vi "VisionTotal.vi"   [LabVIEW 2016]
uses:
  Robot Global Data.vi
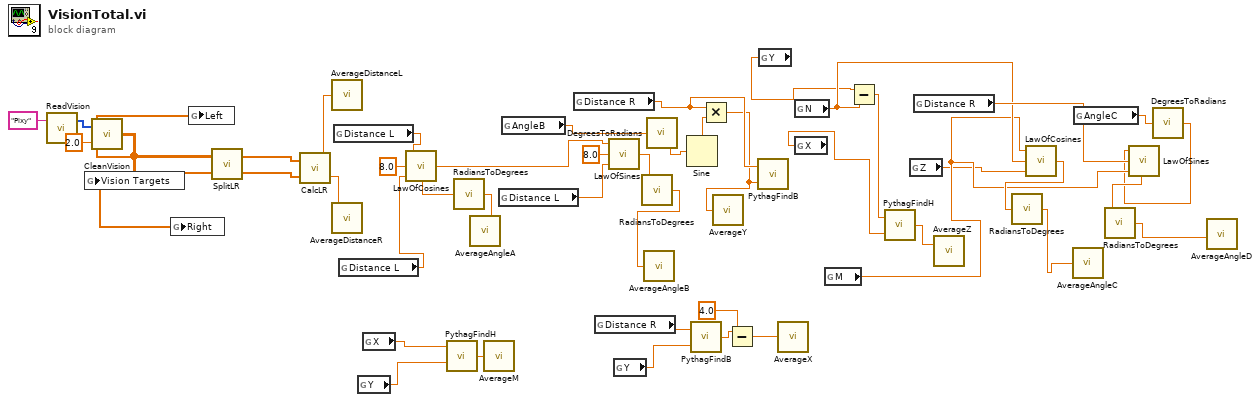
[diagram p0: block diagram]
diagram:
  n1 = call "ReadVision.vi"("Name"="Pixy") -> ("Target Data"=w42:u16[])  [unwired: 2 in]
  n2 = call "CleanVision.vi"("Targets"=2.0, "Input"=w42) -> ("Output"=w41:dbl[][])
  n3 = global write "Robot Global Data.vi" "Vision Targets"(w41) -> ()
  n4 = call "SplitLR.vi"("Vision Targets"=w41) -> ("Right"=w39:dbl[], "Left"=w40:dbl[])  [unwired: 1 in]
  n5 = global write "Robot Global Data.vi" "Right"(w39) -> ()
  n6 = global write "Robot Global Data.vi" "Left"(w40) -> ()
  n7 = call "CalcLR.vi"("Right"=w39, "Left"=w40) -> ("Right"=w25:dbl, "Left"=w24:dbl)
  n8 = call "AverageDistanceL.vi"("Input"=w24) -> ()  [unwired: 1 in]
  n9 = call "AverageDistanceR.vi"("Input"=w25) -> ()  [unwired: 1 in]
  n10 = global read "Robot Global Data.vi" "Distance L"() -> (w12:dbl)
  n11 = global read "Robot Global Data.vi" "Distance L"() -> (w11:dbl)
  n12 = global read "Robot Global Data.vi" "Y"() -> (w1:dbl)
  n13 = global read "Robot Global Data.vi" "X"() -> (w2:dbl)
  n14 = call "LawOfCosines.vi"("Right"=w11, "Opposite"=8.0, "Left"=w12) -> ("Angle"=w35:dbl)
  n15 = call "PythagFindH.vi"("Side B"=w1, "Side A"=w2) -> ("Side H"=w3:dbl)
  n16 = call "RadiansToDegrees.vi"("Radians"=w35) -> ("Degrees"=w23:dbl)
  n17 = call "AverageAngleA.vi"("Input"=w23) -> ()  [unwired: 1 in]
  n18 = call "AverageM.vi"("Input"=w3) -> ()  [unwired: 1 in]
  n19 = global read "Robot Global Data.vi" "Distance L"() -> (w37:dbl)
  n20 = global read "Robot Global Data.vi" "AngleB"() -> (w22:dbl)
  n21 = global read "Robot Global Data.vi" "Distance R"() -> (w34:dbl)
  n22 = global read "Robot Global Data.vi" "Distance R"() -> (w8:dbl)
  n23 = call "LawOfSines.vi"("Opposite Unknown Angle"=w37, "Opposite Known Angle"=8.0, "Known Angle"=w35) -> ("Unknown Angle"=w29:dbl)
  n24 = global read "Robot Global Data.vi" "Y"() -> (w7:dbl)
  n25 = call "RadiansToDegrees.vi"("Radians"=w29) -> ("Degrees"=w13:dbl)
  n26 = call "AverageAngleB.vi"("Input"=w13) -> ()  [unwired: 1 in]
  n27 = call "DegreesToRadians.vi"("Degrees"=w22) -> ("Radians"=w21:dbl)
  n28 = Sine(x=w21) -> (sin(x)=w28:dbl)
  n29 = call "PythagFindB.vi"("Side B"=w7, "Side H"=w8) -> ("Side B"=w6:dbl)
  n30 = Multiply(x=w34, y=w28) -> (x*y=w19:dbl)
  n31 = call "AverageY.vi"("Input"=w19) -> ()  [unwired: 1 in]
  n32 = Subtract(x=w6, y=4.0) -> (x-y=w5:dbl)
  n33 = call "PythagFindB.vi"("Side B"=w19, "Side H"=w34) -> ()  [unwired: 1 out]
  n34 = global read "Robot Global Data.vi" "Y"() -> (w20:dbl)
  n35 = call "AverageX.vi"("Input"=w5) -> ()  [unwired: 1 in]
  n36 = global read "Robot Global Data.vi" "N"() -> (w27:dbl)
  n37 = global read "Robot Global Data.vi" "X"() -> (w32:dbl)
  n38 = global read "Robot Global Data.vi" "M"() -> (w17:dbl)
  n39 = Subtract(x=w20, y=w27) -> (x-y=w33:dbl)
  n40 = call "PythagFindH.vi"("Side B"=w32, "Side A"=w33) -> ("Side H"=w18:dbl)
  n41 = global read "Robot Global Data.vi" "Z"() -> (w14:dbl)
  n42 = global read "Robot Global Data.vi" "Distance R"() -> (w31:dbl)
  n43 = call "AverageZ.vi"("Input"=w18) -> ()  [unwired: 1 in]
  n44 = call "LawOfCosines.vi"("Right"=w14, "Opposite"=w27, "Left"=w17) -> ("Angle"=w26:dbl)
  n45 = call "RadiansToDegrees.vi"("Radians"=w26) -> ("Degrees"=w16:dbl)
  n46 = call "AverageAngleC.vi"("Input"=w16) -> ()  [unwired: 1 in]
  n47 = global read "Robot Global Data.vi" "AngleC"() -> (w10:dbl)
  n48 = call "DegreesToRadians.vi"("Degrees"=w10) -> ("Radians"=w9:dbl)
  n49 = call "LawOfSines.vi"("Opposite Unknown Angle"=w17, "Opposite Known Angle"=w31, "Known Angle"=w9) -> ("Unknown Angle"=w30:dbl)
  n50 = call "RadiansToDegrees.vi"("Radians"=w30) -> ("Degrees"=w15:dbl)
  n51 = call "AverageAngleD.vi"("Input"=w15) -> ()  [unwired: 1 in]
